vi "Turn on, Test, and Turn off Tubes SubVI.vi"(6 "Begin Tube #":i32, 7 "End Tube #":i32, 8 "Clear Pin in":refnum<k21>[](array[refnum]), 9 "Write Pin in":refnum<k21>[](array[refnum]), 10 "Sync Pin in":refnum<k21>[](array[refnum]), 11 "Data Pin in":refnum<k21>[](array[refnum])) -> (0 "Clear Pin out":refnum<k21>, 1 "Write Pin out":refnum<k21>, 2 "Sync Pin out":refnum<k21>, 3 "Data Pin out":refnum<k21>)   [LabVIEW 2020]
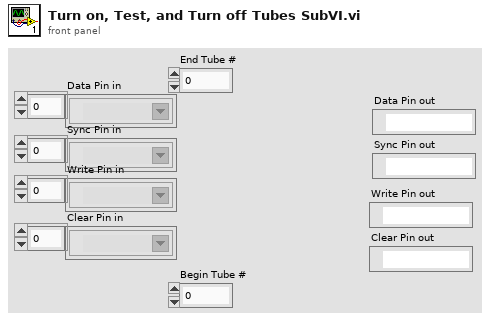
[diagram p1: front panel]
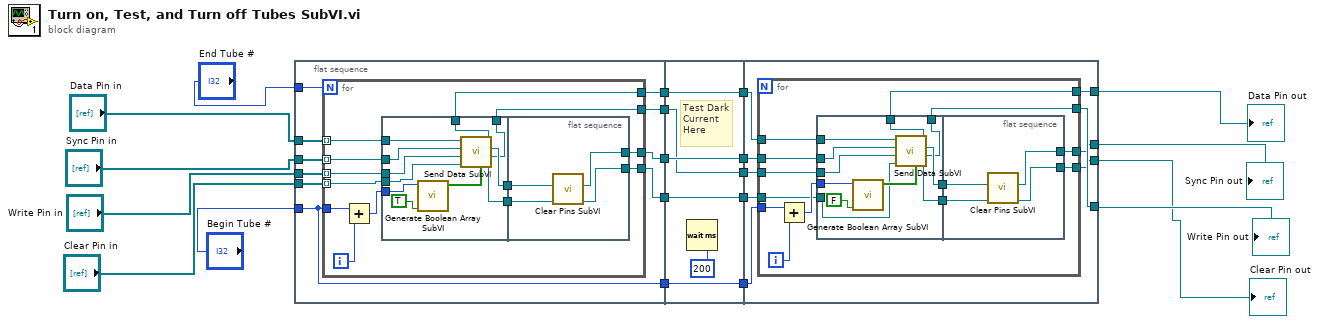
[diagram p0: block diagram]
diagram:
  n1 = flat-sequence {
    tunnel: "Begin Tube #" -> [w27]
    tunnel: "End Tube #" -> [w22]
    tunnel: "Data Pin in" -> [w30]
    tunnel: "Sync Pin in" -> [w29]
    tunnel: "Write Pin in" -> [w28]
    tunnel: [w27] -> w20
    tunnel: [w26] -> w19
    tunnel: [w25] -> w18
    tunnel: [w24] -> w17
    tunnel: [w23] -> w16
    tunnel: "Clear Pin in" -> [w21]
    tunnel: w20 -> [w63]
    tunnel: [w63] -> w15
    tunnel: [w62] -> w14
    tunnel: w19 -> [w62]
    tunnel: [w61] -> w13
    tunnel: w18 -> [w61]
    tunnel: [w60] -> w12
    tunnel: w17 -> [w60]
    tunnel: [w59] -> w11
    tunnel: w16 -> [w59]
    tunnel: w15 -> [w73]
    tunnel: w14 -> [w72]
    tunnel: w13 -> [w71]
    tunnel: w12 -> [w70]
    tunnel: w11 -> [w69]
    tunnel: [w68] -> w5
    tunnel: [w67] -> w4
    tunnel: [w66] -> w3
    tunnel: [w65] -> w2
    frame #0 {
      n2 = for {
        N: w22 -> [_]
        tunnel: w30 -> [w43] mode=indexing
        tunnel: w29 -> [w42] mode=indexing
        tunnel: w28 -> [w41] mode=indexing
        tunnel: [w38] -> w25
        tunnel: [w37] -> w23
        tunnel: [w36] -> w24
        tunnel: [w35] -> w26
        tunnel: w27 -> [w32]
        tunnel: w21 -> [w31] mode=indexing
        i -> [w33]
        n3 = Add(x=w32, y=w33) -> (x+y=w34:i32)
        n4 = flat-sequence {
          tunnel: w34 -> [w52]
          tunnel: w43 -> [w51]
          tunnel: w42 -> [w50]
          tunnel: w41 -> [w49]
          tunnel: [w48] -> w40
          tunnel: [w47] -> w39
          tunnel: [w46] -> w36
          tunnel: [w45] -> w35
          tunnel: w31 -> [w44]
          tunnel: w40 -> [w58]
          tunnel: w39 -> [w57]
          tunnel: [w56] -> w38
          tunnel: [w55] -> w37
          frame #0 {
            n5 = call "Generate Boolean Array SubVI.vi"("Activate: 1\nDeactivate: 0"=TRUE, "Tube"=w52) -> ("Boolean array"=w53:bool[])  [unwired: 9 in]
            n6 = call "Send Data SubVI.vi"("Data Pin Task In"=w51, "Sync Pin Task In"=w50, "Write Pin Task In"=w49, "Clear Pin Task In"=w44, "Data"=w53) -> ("Data Pin Task Out"=w45:refnum<k21>, "Sync Pin Task Out"=w48:refnum<k21>, "Write Pin Task Out"=w46:refnum<k21>, "Clear Pin Task Out"=w47:refnum<k21>)  [unwired: 1 in]
          }
          frame #1 {
            n7 = call "Clear Pins SubVI.vi"("Clear Pin Task In"=w57, "Sync Pin Task In"=w58) -> ("Clear Pin Task Out"=w55:refnum<k21>, "Sync Pin Task Out"=w56:refnum<k21>)  [unwired: 8 in]
          }
        }
      }
    }
    frame #1 {
      # "Test Dark\nCurrent\nHere"
      n8 = Wait (ms)(milliseconds to wait=u32 200) -> ()  [unwired: 1 out]
    }
    frame #2 {
      n9 = for {
        tunnel: w72 -> [w86]
        tunnel: w71 -> [w85]
        tunnel: w70 -> [w84]
        tunnel: [w81] -> w66
        tunnel: [w80] -> w65
        tunnel: [w79] -> w67
        tunnel: [w78] -> w68
        tunnel: w73 -> [w75]
        tunnel: w69 -> [w74]
        i -> [w76]
        n10 = Add(x=w75, y=w76) -> (x+y=w77:i32)
        n11 = flat-sequence {
          tunnel: w77 -> [w95]
          tunnel: w86 -> [w94]
          tunnel: w85 -> [w93]
          tunnel: w84 -> [w92]
          tunnel: [w91] -> w83
          tunnel: [w90] -> w82
          tunnel: [w89] -> w79
          tunnel: [w88] -> w78
          tunnel: w74 -> [w87]
          tunnel: w83 -> [w101]
          tunnel: w82 -> [w100]
          tunnel: [w99] -> w81
          tunnel: [w98] -> w80
          frame #0 {
            n12 = call "Generate Boolean Array SubVI.vi"("Activate: 1\nDeactivate: 0"=FALSE, "Tube"=w95) -> ("Boolean array"=w96:bool[])  [unwired: 9 in]
            n13 = call "Send Data SubVI.vi"("Data Pin Task In"=w94, "Sync Pin Task In"=w93, "Write Pin Task In"=w92, "Clear Pin Task In"=w87, "Data"=w96) -> ("Data Pin Task Out"=w88:refnum<k21>, "Sync Pin Task Out"=w91:refnum<k21>, "Write Pin Task Out"=w89:refnum<k21>, "Clear Pin Task Out"=w90:refnum<k21>)  [unwired: 1 in]
          }
          frame #1 {
            n14 = call "Clear Pins SubVI.vi"("Clear Pin Task In"=w100, "Sync Pin Task In"=w101) -> ("Clear Pin Task Out"=w98:refnum<k21>, "Sync Pin Task Out"=w99:refnum<k21>)  [unwired: 8 in]
          }
        }
      }
    }
  }
  "Data Pin out" <- w5
  "Sync Pin out" <- w3
  "Write Pin out" <- w4
  "Clear Pin out" <- w2
